vi "Set Time.vi"(6 "Second":i32 min=0 max=59 step=1, 7 "Hour":i32 min=0 max=24 step=1, 8 "error in (no error)":errorcluster, 9 "Minute":i32 min=0 max=59 step=1, 10 "Address (0)":i32, 11 "VISA resource name":refnum<visa-resource-name>) -> (0 "error out":errorcluster, 3 "VISA resource name out":refnum<visa-resource-name>)   [LabVIEW 2016, in "Environment Chamber.lvlib" / "Climatic Chamber.lvlib"]
doc: "<b>Time setting</B>\n\nChanges the time of the internal calendar."
uses:
  Climatic Chamber.lvlib
panel:
  out "NACK":bool
  out "Error":bool
  out "ACK":bool
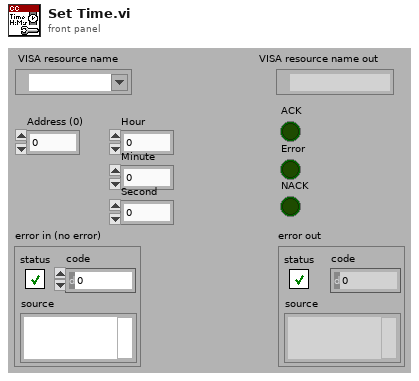
[diagram p1: front panel]
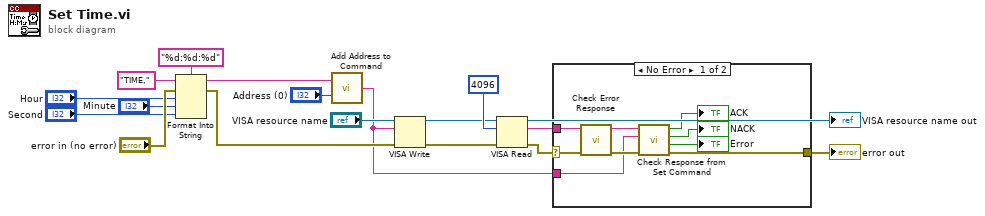
[diagram p0: block diagram]
diagram:
  n1 = Format Into String(format string="%d:%d:%d", initial string="TIME,", error in="error in (no error)", "Hour", "Minute", "Second") -> (resulting string=w4:string, error out=w3:errorcluster)
  n2 = call "Add Address to Command.vi"("Address (0)"="Address (0)", "Command"=w4) -> ("Command OUT"=w2:string)
  n3 = VISA Write(VISA resource name="VISA resource name", write buffer=w2, error in (no error)=w3) -> (VISA resource name out=w15:refnum<visa-resource-name>, error out=w14:errorcluster)  [unwired: 1 out]
  n4 = VISA Read(VISA resource name=w15, byte count=u32 4096, error in (no error)=w14) -> (VISA resource name out=→"VISA resource name out":refnum<visa-resource-name>, read buffer=w10:string, error out=w11:errorcluster)  [unwired: 1 out]
  n5 = case shown="No Error" w11 {
    selector: w11 -> [w26 w28]
    tunnel: w10 -> [w27 _]
    tunnel: [w22 w28] -> w9
    tunnel: w2 -> [w23 _]
    frame No Error {
      n6 = call "Check Error Response.vi"("error in (no error)"=w26, "read String"=w27) -> ("error out"=w25:errorcluster, "String out"=w24:string)  [unwired: 7 in, 1 out]
      n7 = call "Check Response from Set Command.vi"("error in (no error)"=w25, "Command"=w23, "Response"=w24) -> ("error out"=w22:errorcluster, "Error"=→"Error":bool, "NACK"=→"NACK":bool, "ACK"=→"ACK":bool)  [unwired: 5 in]
    }
    frame Error {
    }
  }
  "error out" <- w9
